vi "save_PDS_data.vi"(0 "file path (dialog if empty)":path, 11 "error in (no error)":errorcluster, 13 "PDS Data In":T1) -> (15 "error out":errorcluster)   [LabVIEW 2023]
uses:
  <vilib>/Utility/file.llb/Write Delimited Spreadsheet (string).vi
  <vilib>/Utility/file.llb/Write Delimited Spreadsheet (DBL).vi
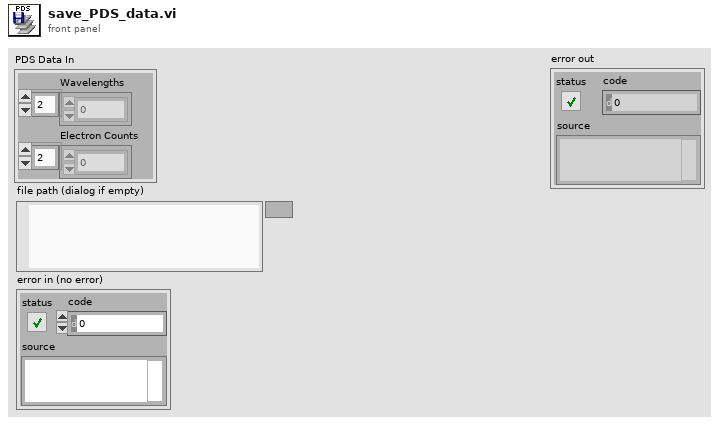
[diagram p1: front panel]
types:
  T1 = cluster{"Wavelengths":dbl[], "Electron Counts":i32[]}
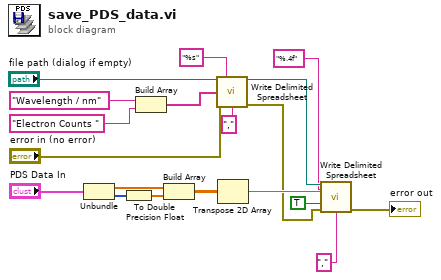
[diagram p0: block diagram]
diagram:
  n1 = Unbundle("PDS Data In") -> ("Wavelengths"=w17:dbl[], "Electron Counts"=w18:i32[])
  n2 = To Double Precision Float(number=w18) -> (double precision float=w16:dbl[])
  n3 = Build Array("Wavelength / nm", "Electron Counts ") -> (w6:string[])
  n4 = Build Array(w17, w16) -> (w15:dbl[][])
  n5 = call-poly <vilib>:"Write Delimited Spreadsheet.vi"("file path (dialog if empty)"="file path (dialog if empty)", "format (%s)"="%s" ("format (%.3f)"), "1D data"=w6, "error in (no error)"="error in (no error)", "delimiter (\\t)"="," ("delimiter (\\t)")) -> ("new file path (Not A Path if cancelled)"=w13:path, "error out"=w12:errorcluster)  [unwired: 9 in]
  n6 = Transpose 2D Array(2D array=w15) -> (transposed array=w14:dbl[][])
  n7 = call-poly <vilib>:"Write Delimited Spreadsheet.vi"("file path (dialog if empty)"=w13, "format (%.3f)"="%.4f", "2D data"=w14, "append to file? (new file:F)"=TRUE, "error in (no error)"=w12, "delimiter (\\t)"="," ("delimiter (\\t)")) -> ("error out"=→"error out":errorcluster)  [unwired: 8 in, 1 out]
